vi "CytecSet.vi"(3 "SwitchMatrix":bool[][](array[boolean]), 4 "VISA resource name":refnum<visa-resource-name>) -> (0 "error out":errorcluster, 1 "VISA resource name out":refnum<visa-resource-name>)   [LabVIEW 2021]
panel:
  in  "error in (no error)":errorcluster
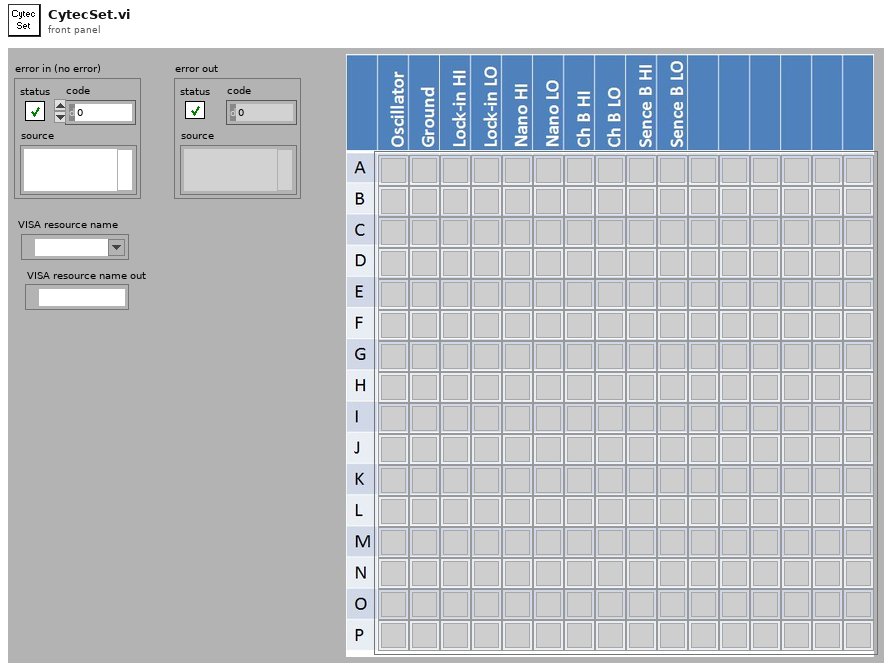
[diagram p1: front panel]
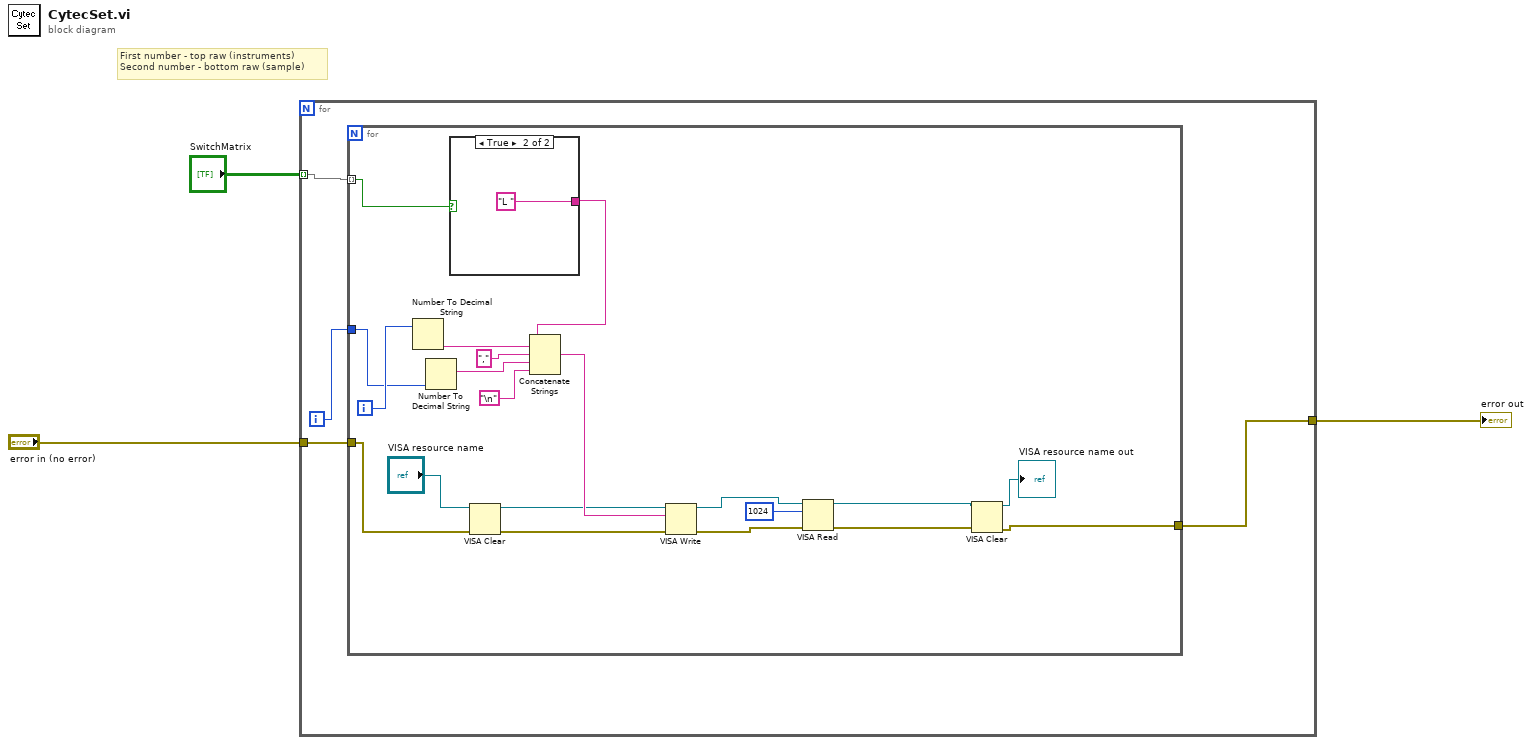
[diagram p0: block diagram]
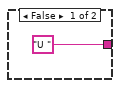
[diagram p2: hidden frame]
diagram:
  # "First number - top raw (instruments)\nSecond number - bottom raw (sample)"
  n1 = for {
    tunnel: [w6] -> w3
    tunnel: "error in (no error)" -> [w5]
    tunnel: "SwitchMatrix" -> [w4] mode=indexing
    i -> [w7]
    n2 = for {
      tunnel: w7 -> [w19]
      tunnel: [w10] -> w6
      tunnel: w5 -> [w14]
      tunnel: w4 -> [w18] mode=indexing
      i -> [w20]
      n3 = Number To Decimal String(number=w20) -> (decimal integer string=w26:string)  [unwired: 1 in]
      n4 = Number To Decimal String(number=w19) -> (decimal integer string=w25:string)  [unwired: 1 in]
      n5 = case shown="True" w18 {
        tunnel: ["U " "L "] -> w27
        frame False {
        }
        frame True {
        }
      }
      n6 = VISA Clear(VISA resource name="VISA resource name", error in (no error)=w14) -> (VISA resource name out=w12:refnum<visa-resource-name>, error out=w13:errorcluster)
      n7 = Concatenate Strings(w27, w26, ",", w25, "\n") -> (w21:string)
      n8 = VISA Write(VISA resource name=w12, write buffer=w21, error in (no error)=w13) -> (VISA resource name out=w17:refnum<visa-resource-name>, error out=w23:errorcluster)  [unwired: 1 out]
      n9 = VISA Read(VISA resource name=w17, byte count=1024, error in (no error)=w23) -> (VISA resource name out=w9:refnum<visa-resource-name>, error out=w11:errorcluster)  [unwired: 2 out]
      n10 = VISA Clear(VISA resource name=w9, error in (no error)=w11) -> (VISA resource name out=→"VISA resource name out":refnum<visa-resource-name>, error out=w10:errorcluster)
    }
  }
  "error out" <- w3
